vi "RT Driver VI.vi"(6 "Device Clock":string, 9 "Device Inputs FIFO":refnum<k33>, 10 "Device Outputs FIFO":refnum<k33>, 11 "Device Reference":T3 format="%.0x") -> ()   [LabVIEW 2021, in "gRPC Data Server Engine.lvlib"]
uses:
  gRPC Data Server Engine.lvlib
  <vilib>/NI VeriStand/Custom Device API/Custom Device Item Ref.ctl
  Shared/Compiled.Settings.ctl
  <vilib>/gRPC/LabVIEW gRPC Library/Shared/grpcId.ctl
  <vilib>/gRPC/LabVIEW gRPC Servicer/Servicer/Servicer.lvclass/Servicer.ctl
  labview-grpc-source/veristand-grpc_server/RPC Service/veristand/veristand-grpc.lvclass
  C:/Program Files/National Instruments/LabVIEW 2021/vi.lib/gRPC/LabVIEW gRPC Servicer/ServiceBase/ServiceBase.lvclass
  labview-grpc-source/veristand-grpc_server/Data/Data Server.lvclass/Data Server.ctl
  <vilib>/NI VeriStand/Custom Device API/Message Response (String).ctl
  <vilib>/NI VeriStand/Custom Device API/Message Response (Byte Array).ctl
  labview-grpc-source/veristand-grpc_server/Data/Data Server.lvclass
  <vilib>/NI VeriStand/Custom Device Tools/Custom Device Utility Library/Custom Device Utility Library.lvlib
  <vilib>/NI VeriStand/Custom Device API/Custom Device API.lvlib
  <vilib>/gRPC/LabVIEW gRPC Servicer/Servicer/Servicer.lvclass
  labview-grpc-source/veristand-grpc_server/Veristandgrpc_server.lvlib
  Shared/gRPC Data Server Shared.lvlib
  <vilib>/gRPC/LabVIEW gRPC Library/grpc-lvsupport-release.lvlib
panel:
  out "error out 2":errorcluster
  out "error out":errorcluster
  out "gRPC ID Out":T1
  out "Settings Out":T2
  in  "Server Settings":T2={"Name"="", "Server Address"="localhost:50051", "Async?"=FALSE, "Key File"=path "", "Cert File"=path "", "Channel Name"=["First Name", "Last Name", "Full Name"], "Initial Value"=["John", "Cena"]}
  in  "Debug Stop":bool
  in  "Debug":bool
  out "Data Loop Iteration":i32
  out "Current Value":string[](array[string])
  out "Listening Port":i32
  in  "Initialization Status Notifier":refnum<notifier>
  in  "Status Notifier":refnum<notifier>
  # "Custom Device Template\nv1.0"
  # "Use this template as a starting point for creating a custom device code module. The input controls shown here are specially named controls that the system will use to provide the device loop with data. The controls are not required for the device loop to run. For instance, if the device doesn't produce any output data, then you don't need the Device Outputs FIFO control. If you do use these controls, however, they need to have these exact names to be functional."
  # "Debug Panel in ADE"
  # "The optional status notifier element is used to notify the RT engine of the last state of the custom device, and to indicate the device has completed execution. If this control is not used, a default No Error value is returned to the system when the device finishes execution.\n\nNote: This error state is not checked until the system shuts down. Use an output status channel to send more immediate status values to the system."
  # "This optional input can be used to send the VeriStand Engine the final status of the custom device initalization process. If this control exists on the custom device front panel, the VeriStand Engine will wait for a status update before starting up. If the custom device reports an error, that will abort the execution of the current configuration in the VeriStand Engine.\n\nThis control can be deleted if the custom device does not need to send the initialization status update."
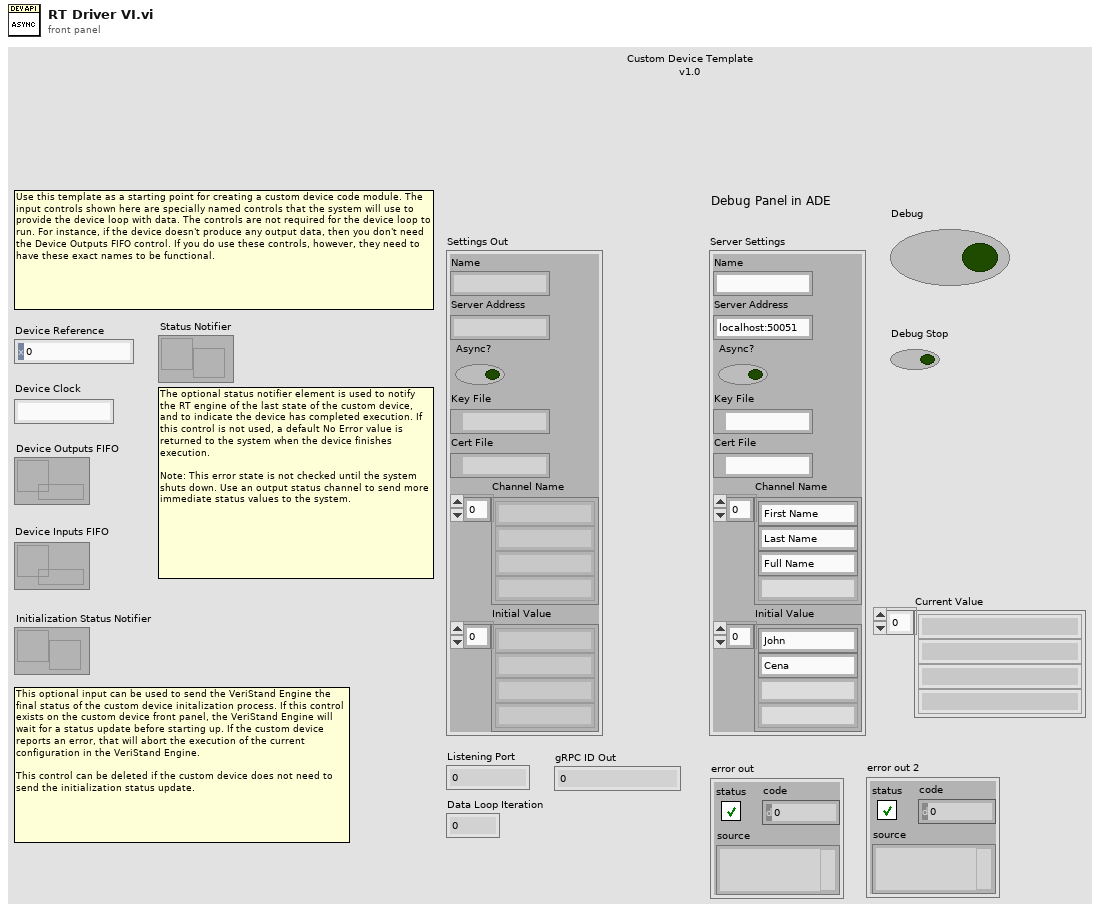
[diagram p1: front panel]
types:
  T1 = typedef "grpc-lvsupport-release.lvlib/grpcId.ctl" = u64
  T2 = typedef "gRPC Data Server Shared.lvlib/Compiled.Settings.ctl" = cluster{"Name":string, "Server Address":string, "Async?":bool, "Key File":path, "Cert File":path, "Channel Name":string[], "Initial Value":string[]}
  T3 = typedef "Custom Device API.lvlib/Custom Device Item Ref.ctl" = u64
  T4 = typedef "Custom Device API.lvlib/Custom Device Engine Event Ref.ctl" = refnum<event-registration>
  T5 = enum32{"Invalid", "Standard", "Closed", "Hidden", "Minimized", "Maximized"}
  T6 = typedef "Custom Device API.lvlib/Message Response (String).ctl" = cluster{"Response":string, "Error":errorcluster}
  T7 = typedef "Custom Device API.lvlib/Message Response (Byte Array).ctl" = cluster{"Response":u8[], "Error":errorcluster}
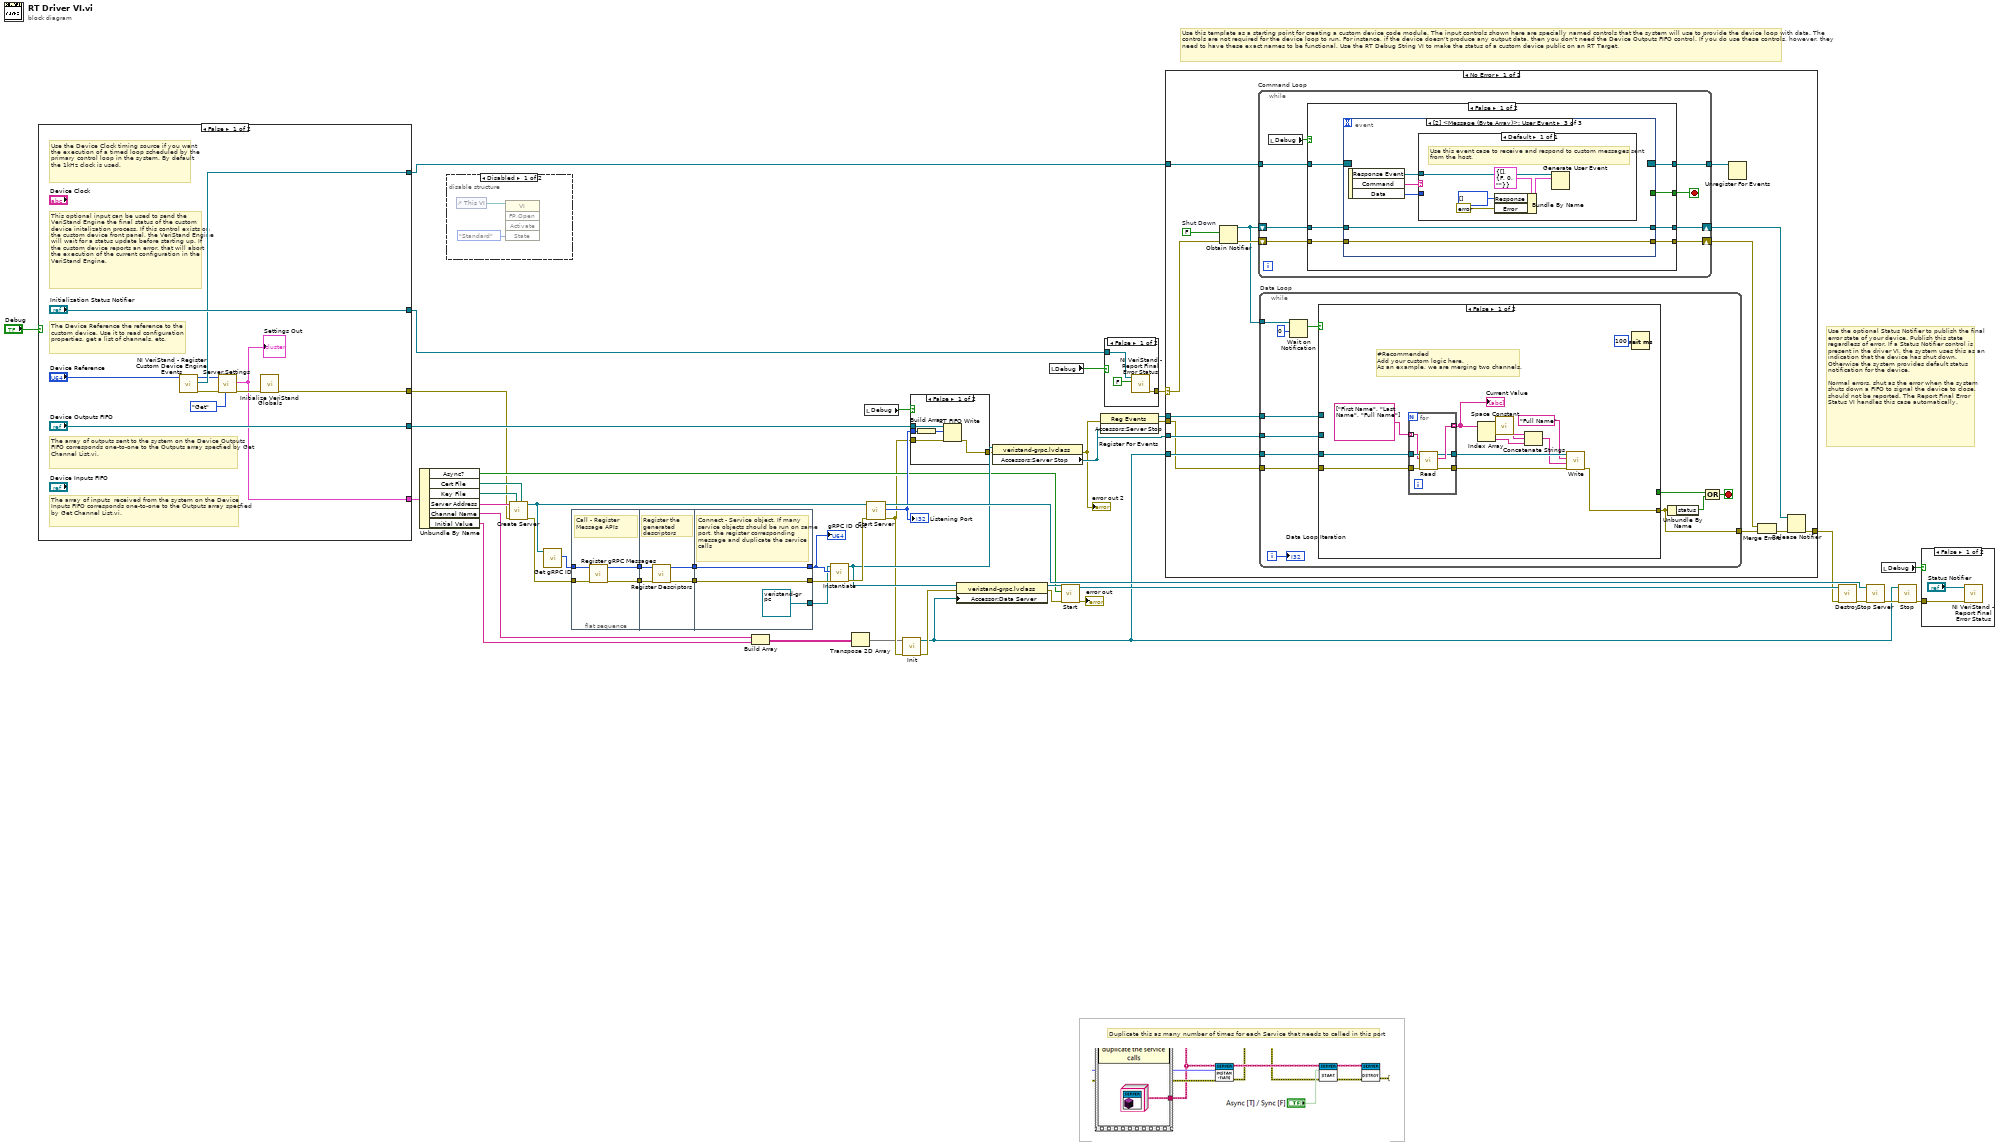
[diagram p0: block diagram]
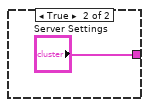
[diagram p6: hidden frame]
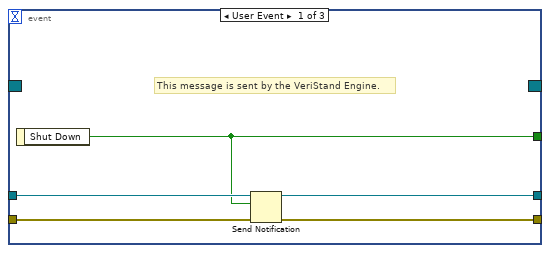
[diagram p7: hidden frame]
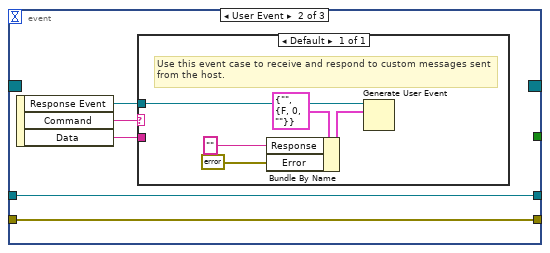
[diagram p8: hidden frame]
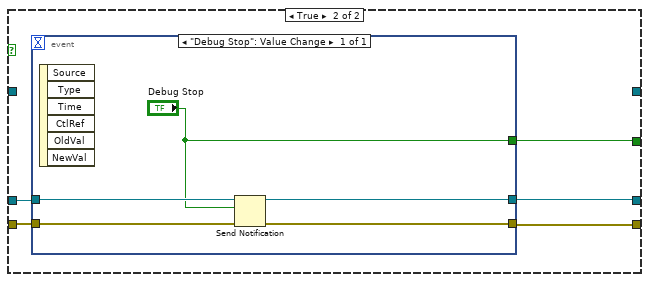
[diagram p9: hidden frame]
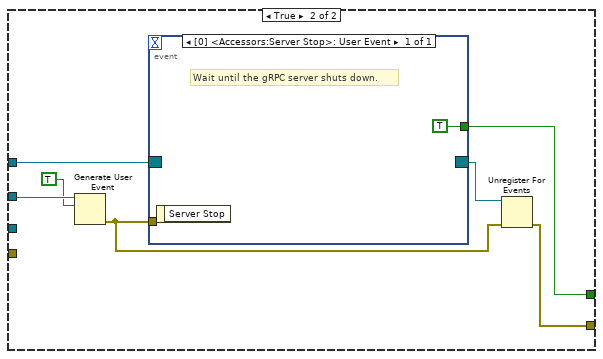
[diagram p10: hidden frame]
diagram:
  # "Duplicate this as many number of times for each Service that needs to called in this port"
  # "Use the optional Status Notifier to publish the final error state of your device. Publish this state regardless of error. If a Status Notifier control is present in the driver VI, the system uses this as an indication that the device has shut down. Otherwise the system provides default status notification for the device.\n\nNormal errors, shut as the error when the system shuts down a FIFO to signal the device to close, should not be reported. The Report Final Error Status VI handles this case automatically."
  # "Use this template as a starting point for creating a custom device code module. The input controls shown here are specially named controls that the system will use to provide the device loop with data. The controls are not required for the device loop to run. For instance, if the device doesn't produce any output data, then you don't need the Device Outputs FIFO control. If you do use these controls, however, they need to have these exact names to be functional. Use the RT Debug String VI to make the status of a custom device public on an RT Target."
  n1 = case shown="False" "Debug" {
    tunnel: ["Initialization Status Notifier" _] -> w48
    tunnel: [w50 "Server Settings"] -> w27
    tunnel: ["Device Outputs FIFO" _] -> w23
    tunnel: [w56 _] -> w18
    tunnel: [w54 _] -> w3
    frame False {
      # "This optional input can be used to send the VeriStand Engine the final status of the custom device initalization process. If this control exists on the custom device front panel, the VeriStand Engine will wait for a status update before starting up. If the custom device reports an error, that will abort the execution of the current configuration in the VeriStand Engine."
      # "The array of inputs  received from the system on the Device Inputs FIFO corresponds one-to-one to the Outputs array specfied by Get Channel List.vi."
      # "The array of outputs sent to the system on the Device Outputs FIFO corresponds one-to-one to the Outputs array specfied by Get Channel List.vi."
      # "The Device Reference the reference to the custom device. Use it to read configuration properties, get a list of channels, etc."
      # "Use the Device Clock timing source if you want the execution of a timed loop scheduled by the primary control loop in the system. By default the 1kHz clock is used."
      n2 = call <vilib>:"NI VeriStand - Register Custom Device Engine Events.vi"("Device Ref in"="Device Reference") -> ("error out"=w52:errorcluster, "Custom Device Engine Event Ref"=w56:T4, "Device Ref out"=w53:T3)  [unwired: 8 in]
      n3 = call "Server.Settings.vi"("Action"=enum8{"Get", "Set"}."Get", "error in (no error)"=w52, "Parent Ref in"=w53) -> ("error out"=w51:errorcluster, "Settings Out"=w50:T2)  [unwired: 6 in, 1 out]
      "Settings Out" <- w50
      n4 = call "Initialize VeriStand Globals.vi"("error in (no error)"=w51) -> ("error out"=w54:errorcluster)  [unwired: 10 in]
    }
    frame True {
    }
  }
  n5 = Unbundle By Name(w27) -> ("Async?"=w19:bool, "Cert File"=w24:path, "Key File"=w25:path, "Server Address"=w26:string, "Channel Name"=w22:string[], "Initial Value"=w21:string[])
  n6 = disable-structure shown="Disabled" {
    frame Disabled {
      n7 = control-ref of="This VI"() -> (w60:refnum<vi>)
      n8 = invoke class="VI" method="FP.Open"(reference=w60, "State"=T5."Standard") -> ()  [unwired: 3 in, 5 out]
    }
    frame Enabled {
    }
  }
  n9 = call <vilib>:"Create Server.vi"("Server Key File (.key)"=w24, "Server Certificate File (.crt)"=w25, "error in"=w3, "Server Address"=w26) -> ("error out"=w37:errorcluster, "gRPC Server out"=w41:refnum<class "Servicer.lvclass">)  [unwired: 6 in]
  n10 = call <vilib>:"Get gRPC ID.vi"("OOP Server in"=w41) -> ("gRPC ID"=w38:T1)  [unwired: 9 in, 1 out]
  n11 = flat-sequence {
    tunnel: w38 -> [w63]
    tunnel: w37 -> [w65]
    tunnel: [w64] -> w46
    tunnel: [w62] -> w45
    tunnel: w46 -> [w68]
    tunnel: w45 -> [w69]
    tunnel: [w66] -> w44
    tunnel: [w67] -> w43
    tunnel: [w71] -> w35
    tunnel: [w72] -> w36
    tunnel: w44 -> [w72]
    tunnel: w43 -> [w71]
    tunnel: [refnum<class "veristand-grpc.lvclass"> refnum ("veristand-grpc_server.lvlib:veristand.lvclass")] -> w33
    frame #0 {
      # "Call - Register Message APIs"
      n12 = call "Register gRPC Messages.vi"("error in (no error)"=w65, "gRPC ID"=w63) -> ("error out"=w64:errorcluster, "gRPC ID Out"=w62:T1)  [unwired: 8 in]
    }
    frame #1 {
      # "Register the generated descriptors"
      n13 = call "Register Descriptors.vi"("error in (no error)"=w68, "gRPC ID"=w69) -> ("error out"=w66:errorcluster, "gRPC ID Out"=w67:T1)  [unwired: 8 in]
    }
    frame #2 {
      # "Connect - Service object. If many service objects should be run on same port, the register corresponding message and duplicate the service calls"
    }
  }
  n14 = Build Array(w22, w21) -> (w9:string[][])
  n15 = call-dynamic "Instantiate.vi"("error in"=w36, "gRPCid"=w35, "iService"=w33) -> ("error out"=w40:errorcluster, "iService"=w32:refnum<class "veristand-grpc.lvclass">)  [unwired: 7 in]
  n16 = Transpose 2D Array(2D array=w9) -> (transposed array=w8:string[][])
  n17 = local read "Debug"() -> (w6:bool)
  n18 = call <vilib>:"Start Server.vi"("error in"=w40, "gRPC Server in"=w41) -> ("error out"=w16:errorcluster, "Listening Port"=w20:i32, "gRPC Server out"=w42:refnum<class "Servicer.lvclass">)  [unwired: 7 in]
  "Listening Port" <- w20
  n19 = call "Init.vi"("error in (no error)"=w16, "Initial Data"=w8) -> ("error out"=w28:errorcluster, "DVR out"=w11:refnum<class "Data Server.lvclass">)  [unwired: 8 in]
  n20 = case shown="False" w6 {
    tunnel: w23 -> [w77 _]
    tunnel: w20 -> [w76 _]
    tunnel: w16 -> [w75 w78]
    tunnel: [w74 w78] -> w15
    frame False {
      n21 = Build Array(w76) -> (w73:i32[])
      n22 = RT FIFO Write(0:w77, 1:w73, 3:w75) -> (11:w74:errorcluster)  [unwired: 1 in, 4 out]
    }
    frame True {
    }
  }
  n23 = property class="veristand-grpc.lvclass"(reference=w32, error in=w28, "Accessor:Data Server"=w11) -> (reference out=w31:refnum<class "veristand-grpc.lvclass">, error out=w30:errorcluster)
  n24 = property class="veristand-grpc.lvclass"(reference=w32, error in=w15) -> (error out=w1:errorcluster, "Accessors:Server Stop"=w17:refnum<user-event>)  [unwired: 1 out]
  "error out 2" <- w1
  n25 = local read "Debug"() -> (w5:bool)
  n26 = call-dynamic "Start.vi"("error in"=w30, "ASync [T]"=w19, "iService in"=w31) -> ("error out"=→"error out":errorcluster, "iService out"=w34:refnum<class "veristand-grpc.lvclass">)  [unwired: 7 in]
  n27 = register-events(error in=w1, w17) -> (reference out=w14:refnum<event-registration>, error out=w10:errorcluster)  [unwired: 1 in]
  n28 = case shown="False" w5 {
    tunnel: w48 -> [w81 _]
    tunnel: [w80 _] -> w47
    frame False {
      n29 = call <vilib>:"NI VeriStand - Report Final Error Status.vi"("Filter FIFO & Shutdown Errors (T)"=FALSE ("Filter FIFO Errors (T)"), "Status Notifier"=w81) -> ("error out"=w80:errorcluster)  [unwired: 1 in, 8 out]
    }
    frame True {
    }
  }
  n30 = case shown="No Error" w47 {
    selector: w47 -> [w89 w186]
    tunnel: w18 -> [w95 _]
    tunnel: [w93 w186] -> w13
    tunnel: w17 -> [w86 _]
    tunnel: w14 -> [w85 _]
    tunnel: w11 -> [w84 _]
    tunnel: w10 -> [w83 _]
    frame No Error {
      w94 = FALSE  # Shut Down
      n31 = Obtain Notifier(notification data type=w94, error in (no error)=w89) -> (notifier out=w91:refnum<notifier>, error out=w96:errorcluster)  [unwired: 2 in, 1 out]
      n32 = while "Command Loop" {
        tunnel: w95 -> [w104]
        tunnel: [w103] -> w92
        shift-right: [w100] -> w90
        shift-left: w91 -> [w101]
        shift-right: [w98] -> w87
        shift-left: w96 -> [w99]
        stop <- w102 stop-if-true
        n33 = local read "Debug"() -> (w97:bool)
        n34 = case shown="False" w97 {
          tunnel: w104 -> [w111 _]
          tunnel: [w110 _] -> w103
          tunnel: [w109 w137] -> w102
          tunnel: w101 -> [w108 w141]
          tunnel: [w107 w139] -> w100
          tunnel: w99 -> [w106 w140]
          tunnel: [w105 w138] -> w98
          frame False {
            n35 = event shown="[2] <Message (Byte Array)>: User Event" {
              selector: w111 -> [_ _ _]
              dyn-events: [_ _ _] -> w110
              timeout: _ -> [_ _ _]
              tunnel: [w114 _ _] -> w109
              tunnel: w108 -> [w115 w119 w129]
              tunnel: [w116 w119 w129] -> w107
              tunnel: w106 -> [w113 w117 w127]
              tunnel: [w112 w117 w127] -> w105
              event User Event {
                # "This message is sent by the VeriStand Engine."
                n36 = event-data() -> ("Shut Down"=w114:bool)  [unwired: 1 in]
                n37 = Send Notification(notification=w114, notifier=w115, error in (no error)=w113) -> (notifier out=w116:refnum<notifier>, error out=w112:errorcluster)
              }
              event User Event {
                n38 = event-data() -> ("Response Event"=w118:refnum<user-event>, "Command"=w121:string, "Data"=w120:string)  [unwired: 1 in]
                n39 = case shown="Default" w121 {
                  tunnel: w120 -> [_]
                  tunnel: w118 -> [w126]
                  frame Default {
                    # "Use this event case to receive and respond to custom messages sent from the host."
                    n40 = Bundle By Name(cluster=T6 {"Response"="", "Error"={"status"=FALSE, "code"=0, "source"=""}} ("event data"), "Response"="", "Error"=errorcluster {"status"=FALSE, "code"=0, "source"=""}) -> (w124:T6)
                    n41 = Generate User Event(user event=w126, event data cluster=w124) -> ()  [unwired: 2 in, 2 out]
                  }
                }
              }
              event User Event {
                n42 = event-data() -> ("Response Event"=w128:refnum<user-event>, "Command"=w131:string, "Data"=w130:u8[])  [unwired: 1 in]
                n43 = case shown="Default" w131 {
                  tunnel: w130 -> [_]
                  tunnel: w128 -> [w136]
                  frame Default {
                    # "Use this event case to receive and respond to custom messages sent from the host."
                    n44 = Bundle By Name(cluster=T7 {"Response"=[], "Error"={"status"=FALSE, "code"=0, "source"=""}} ("event data"), "Response"=u8[] [], "Error"=errorcluster {"status"=FALSE, "code"=0, "source"=""}) -> (w133:T7)
                    n45 = Generate User Event(user event=w136, event data cluster=w133) -> ()  [unwired: 2 in, 2 out]
                  }
                }
              }
            }
          }
          frame True {
            n46 = event shown="[0] \"Debug Stop\": Value Change" {
              selector: _ -> [_]
              dyn-events: _ -> [_]
              timeout: _ -> [_]
              tunnel: w141 -> [w146]
              tunnel: ["Debug Stop"] -> w137
              tunnel: [w144] -> w139
              tunnel: [w143] -> w138
              tunnel: w140 -> [w142]
              event "Debug Stop": Value Change {
                n47 = event-data() -> ()  [unwired: 1 in, 6 out]
                n48 = Send Notification(notification="Debug Stop", notifier=w146, error in (no error)=w142) -> (notifier out=w144:refnum<notifier>, error out=w143:errorcluster)
              }
            }
          }
        }
      }
      n49 = while "Data Loop" {
        tunnel: w91 -> [w157]
        tunnel: w86 -> [w153]
        tunnel: w85 -> [w152]
        tunnel: w84 -> [w150]
        tunnel: w83 -> [w149]
        tunnel: [w148] -> w82
        i -> [w147]
        stop <- w154 stop-if-true
        n50 = Wait on Notification(notifier=w157, timeout in ms (-1)=0) -> (notification=w156:bool)  [unwired: 2 in, 3 out]
        n51 = case shown="False" w156 {
          tunnel: [_ w181] -> w155
          tunnel: w153 -> [_ w183]
          tunnel: w152 -> [_ w184]
          tunnel: w150 -> [w170 _]
          tunnel: w149 -> [w169 _]
          tunnel: [w159 w178] -> w148
          frame False {
            # "#Recommended\nAdd your custom logic here.\nAs an example, we are merging two channels."
            n52 = for {
              tunnel: w170 -> [w177]
              tunnel: w169 -> [w176]
              tunnel: string[] ["First Name", "Last Name", "Full Name"] -> [w175] mode=indexing
              tunnel: [w174] -> w167 mode=indexing
              tunnel: [w173] -> w163
              tunnel: [w172] -> w162
              n53 = call "Read.vi"("error in (no error)"=w176, "Channel Name"=w175, "Data in"=w177) -> ("error out"=w172:errorcluster, "Data"=w174:string, "Data out"=w173:refnum<class "Data Server.lvclass">)  [unwired: 5 in, 1 out]
            }
            "Current Value" <- w167
            n54 = Index Array(array=w167) -> (element #1=w166:string, element #2=w164:string)  [unwired: 2 in]
            n55 = call <vilib>:"Space Constant.vi"() -> ("String"=w165:string)
            n56 = Concatenate Strings(w166, w165, w164) -> (w161:string)
            n57 = call "Write.vi"("error in (no error)"=w162, "New Data"=w161, "Channel Name"="Full Name", "Data in"=w163) -> ("error out"=w159:errorcluster)  [unwired: 5 in, 2 out]
            n58 = Wait (ms)(milliseconds to wait=u32 100) -> ()  [unwired: 1 out]
          }
          frame True {
            n59 = Generate User Event(user event=w183, event data cluster=TRUE ("event data")) -> (error out=w179:errorcluster)  [unwired: 2 in, 1 out]
            n60 = event shown="[0] <Accessors:Server Stop>: User Event" {
              selector: w184 -> [_]
              dyn-events: [_] -> w180
              timeout: _ -> [_]
              tunnel: [TRUE] -> w181
              tunnel: w179 -> [_]
              event User Event {
                # "Wait until the gRPC server shuts down."
                n61 = event-data() -> ()  [unwired: 1 in, 1 out]
              }
            }
            n62 = Unregister For Events(event registration refnum=w180, error in=w179) -> (error out=w178:errorcluster)
          }
        }
        n63 = Unbundle By Name(w148) -> ("status"=w151:bool)
        n64 = Compound Arithmetic op=OR(w155, w151) -> (w154:bool)
        "Data Loop Iteration" <- w147
      }
      n65 = Unregister For Events(event registration refnum=w92) -> ()  [unwired: 1 in, 1 out]
      n66 = Merge Errors(w87, w82) -> (w88:errorcluster)
      n67 = Release Notifier(notifier=w90, error in (no error)=w88) -> (error out=w93:errorcluster)  [unwired: 1 in, 2 out]
    }
    frame Error {
    }
  }
  n68 = call-dynamic "Destroy.vi"("error in (no error)"=w13, "SignalGeneratorService in"=w34) -> ("error out"=w39:errorcluster)  [unwired: 8 in, 1 out]
  n69 = call <vilib>:"Stop Server.vi"("error in"=w39, "gRPC Server in"=w42) -> ("error out"=w29:errorcluster)  [unwired: 9 in]
  n70 = local read "Debug"() -> (w4:bool)
  n71 = call "Stop.vi"("error in (no error)"=w29, "DVR in"=w11) -> ("error out"=w12:errorcluster)  [unwired: 9 in]
  n72 = case shown="False" w4 {
    tunnel: w12 -> [w188 _]
    frame False {
      n73 = call <vilib>:"NI VeriStand - Report Final Error Status.vi"("error in (no error)"=w188, "Status Notifier"="Status Notifier") -> ()  [unwired: 1 in, 9 out]
    }
    frame True {
    }
  }
  "gRPC ID Out" <- w35
